vi "add gated region to graph.vi"(9 "image in":dbl[][](array[numeric]), 11 "which gate":u16(ring) items=["pulser", "gate 1", "gate 2", "gate 3", "none"]) -> (1 "image out":dbl[][](array[numeric]), 2 "X name output 2":string, 3 "X name output":string)   [LabVIEW 2016]
panel:
  in  "error in (no error)":errorcluster
  out "error out":errorcluster
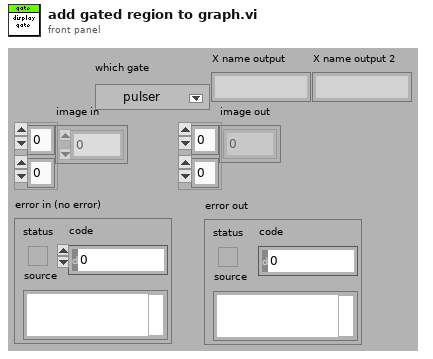
[diagram p1: front panel]
types:
  T1 = typedef "energy 2d selection.ctl" = string
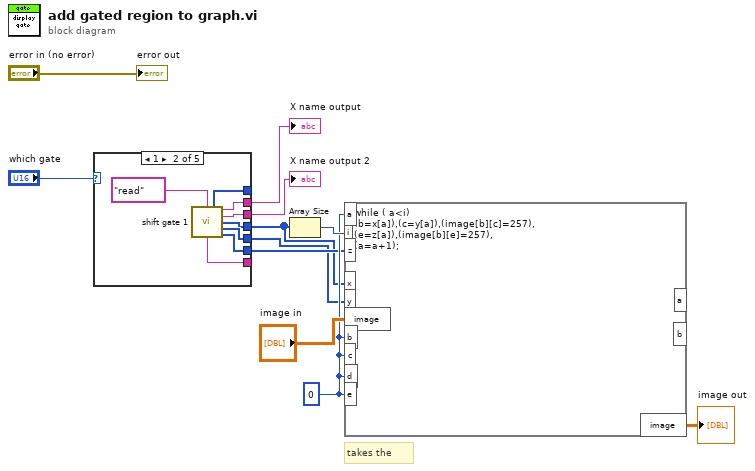
[diagram p0: block diagram]
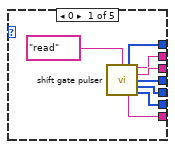
[diagram p2: hidden frame]
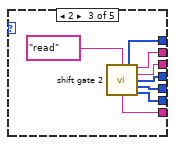
[diagram p3: hidden frame]
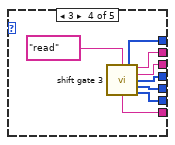
[diagram p4: hidden frame]
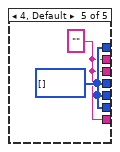
[diagram p5: hidden frame]
diagram:
  w8 = 0 ("input variable")
  # "takes the"
  n1 = case shown="1" "which gate" {
    tunnel: [w19 w27 w35 w43 w44] -> w1
    tunnel: [w18 w26 w28 w36 w44] -> _
    tunnel: [w17 w25 w34 w42 w44] -> w2
    tunnel: [w16 w24 w33 w41 w45] -> w5
    tunnel: [w15 w23 w32 w40 w45] -> w3
    tunnel: [w14 w22 w31 w39 w45] -> w4
    tunnel: [w12 w20 w29 w37 w45] -> _
    frame 0 {
      n2 = call "shift gate pulser.vi"("shift control"="read") -> ("2d array width output"=w12:i32[], "X name output"=w17:string, "Y name  output"=w19:string, "X range output"=w14:i32[], "Y range Max output"=w15:i32[], "Energy 2d gate out"=w18:T1, "Y range Min output"=w16:i32[])  [unwired: 8 in]
    }
    frame 1 {
      n3 = call "shift gate 1.vi"("shift control"="read") -> ("2d  array width output"=w20:i32[], "X name output"=w25:string, "Y name  output"=w27:string, "X range output"=w22:i32[], "Y range Max output"=w23:i32[], "Energy 2d gate out"=w26:T1, "Y range Min output"=w24:i32[])  [unwired: 8 in]
    }
    frame 2 {
      n4 = call "shift gate 2.vi"("shift control"="read") -> ("2d position array output"=w29:i32[], "X name output"=w34:string, "Y name  output"=w35:string, "X range output"=w31:i32[], "Y range Max output"=w32:i32[], "Energy 2d gate out"=w28:T1, "Y range Min output"=w33:i32[])  [unwired: 8 in]
    }
    frame 3 {
      n5 = call "shift gate 3.vi"("shift control"="read") -> ("2d location array output"=w37:i32[], "X name output"=w42:string, "Y name  output"=w43:string, "X range output"=w39:i32[], "Y range Max output"=w40:i32[], "Energy 2d gate out"=w36:T1, "Y range Min output"=w41:i32[])  [unwired: 8 in]
    }
    frame 4, Default {
      w45 = i32[] [] ("X range output")
      w44 = "" ("X name output")
    }
  }
  "X name output" <- w2
  "X name output 2" <- w1
  n6 = Array Size(array=w4) -> (size(s)=w9:i32)
  n7 = formula code="while ( a<i)\n(b=x[a]),(c=y[a]),(image[b][c]=257),\n(e=z[a]),(image[b][e]=257),\n(a=a+1);"("x"=w4, "y"=w3, "image"="image in", "i"=w9, "a"=w8, "b"=w8, "c"=w8, "d"=w8, "e"=w8, "z"=w5) -> ("image"=→"image out":dbl[][])  [unwired: 2 out]
  "error out" <- "error in (no error)"
